vi "Main.vi"(10 "Monedas Subpanel":refnum<vi>, 11 "Module Admin":refnum<class "Delacor_lib_QMH_Module Admin.lvclass">) -> ()   [LabVIEW 2020, in "Monedas.lvlib"]
doc: "This template is based off of the Queued Message Handler design pattern and the Queued Message Handler project template that ships with LabVIEW.\n\nThe main difference is that the queue is private to this module and communication between modules is performed via Broadcast and Request events.\n\nRequest events are wrapped in public API methods and are handled in the Event Handling Loop (EHL) of this VI. Any module can register for Broadcast events sent by this module. The EHL generates messages based on user interface actions.\n\nThe Message Handling Loop (MHL) processes messages generated by the EHL, or by other messages. The messages are string values, so new messages can be added easily to the Message Cases case structure in the MHL. Each message cluster can also provide an optional value for Message Data, which is a variant that can be converted to whatever message-specific data is required.\n_____\nBased on Delacor QMH Project Template 5.0.0.82."
uses:
  Monedas.lvlib
  <vilib>/Delacor/Delacor QMH/Libraries/Module Admin_class/Delacor_lib_QMH_Module Admin.lvclass
  Module Data--cluster.ctl
  Type defMonedasread.ctl
  Stop Argument--cluster.ctl
  <vilib>/Delacor/Delacor QMH/Libraries/Message Queue_class/Delacor_lib_QMH_Message Queue.lvclass/Delacor_lib_QMH_Message Queue.ctl
  <vilib>/Delacor/Delacor QMH/Libraries/Module Admin_class/Delacor_lib_QMH_Module Admin.lvclass/Delacor_lib_QMH_Module Admin.ctl
  botones uno, dos, tres, cuatro Argument--cluster.ctl
  Set Coins Valuessssss Argument--cluster.ctl
  <vilib>/Utility/miscctls.llb/LVPointTypeDef.ctl
  <vilib>/Delacor/Delacor QMH/Libraries/Message Queue_class/Delacor_lib_QMH_Enqueue Message (Single).vi
  <vilib>/Delacor/Delacor QMH/Libraries/Module Admin_class/Delacor_lib_QMH_Get External Launch.vi
  <vilib>/Utility/error.llb/Error Cluster From Error Code.vi
  <vilib>/ErrorRing/Error Ring.xnode
  <vilib>/Delacor/Delacor QMH/Libraries/Message Queue_class/Delacor_lib_QMH_Message Queue.lvclass
  Mensajes/Mensajes.lvlib
  Config/Config.lvlib
  Producto/Producto.lvlib
panel:
  out "Valores monedas":dbl
  in  "Monedas cluster":T1
  out "error out":errorcluster
  out "Status":string
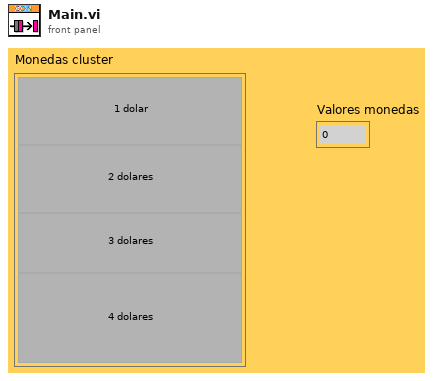
[diagram p1: front panel]
types:
  T1 = cluster{"1 cash":bool, "2 cash":bool, "3 cash":bool, "4 cash ":bool}
  T2 = typedef "Producto.lvlib/Broadcast Events--cluster.ctl" = cluster{"Module Did Init":refnum<user-event>, "Status Updated":refnum<user-event>, "Error Reported":refnum<user-event>, "Module Did Stop":refnum<user-event>, "Update Module Execution Status":refnum<user-event>}
  T3 = typedef "Mensajes.lvlib/Broadcast Events--cluster.ctl" = cluster{"Module Did Init":refnum<user-event>, "Status Updated":refnum<user-event>, "Error Reported":refnum<user-event>, "Module Did Stop":refnum<user-event>, "Update Module Execution Status":refnum<user-event>}
  T4 = typedef "Config.lvlib/Broadcast Events--cluster.ctl" = cluster{"Module Did Init":refnum<user-event>, "Status Updated":refnum<user-event>, "Error Reported":refnum<user-event>, "Module Did Stop":refnum<user-event>, "Update Module Execution Status":refnum<user-event>}
  T5 = typedef "Monedas.lvlib/Request Events--cluster.ctl" = cluster{"Stop Module":refnum<user-event>, "Show Panel":refnum<user-event>, "Hide Panel":refnum<user-event>, "Get Module Execution Status":refnum<user-event>, "Show Diagram":refnum<user-event>, "botones uno, dos, tres, cuatro":refnum<user-event>, "Set Coins Valuessssss":refnum<user-event>}
  T6 = typedef "Monedas.lvlib/Module Data--cluster.ctl" = cluster{"Status":string, "Coins":T7, "Monedas cluster":cluster{"1 cash":bool, "2 cash":bool, "3 cash":bool, "4 cash ":bool}, "Valores monedas":dbl, "refs":cluster{"Reference boton 1":refnum<vi>, "Reference boton 2":refnum<vi>, "Reference boton 3":refnum<vi>, "Reference boton 4":refnum<vi>}}
  T7 = typedef "Type defMonedasread.ctl" = cluster{"Boolean Text":string, "Value":dbl}[]
  T8 = enum32{"invalid lock state", "Not Locked", "Locked (No Password)", "Password-protected"}
  T9 = typedef "Monedas.lvlib/Stop Argument--cluster.ctl" = cluster{"Origin":string, "Exit via Stop Module Req?":bool, "Wait for Module to stop?":bool}
  T10 = typedef "Monedas.lvlib/botones uno, dos, tres, cuatro Argument--cluster.ctl" = cluster{"Monedas cluster":cluster{"1 cash":bool, "2 cash":bool, "3 cash":bool, "4 cash ":bool}}
  T11 = typedef "Monedas.lvlib/Set Coins Valuessssss Argument--cluster.ctl" = cluster{"COINS":cluster{"Boolean Text":string, "Numeric":dbl}[]}
  T12 = typedef "LVPointTypeDef.ctl" = cluster{"Horizontal":i16, "Vertical":i16}
  T13 = enum32{"Invalid", "Standard", "Closed", "Hidden", "Minimized", "Maximized"}
  T14 = cluster{"Reference boton 1":refnum<vi>, "Reference boton 2":refnum<vi>, "Reference boton 3":refnum<vi>, "Reference boton 4":refnum<vi>}
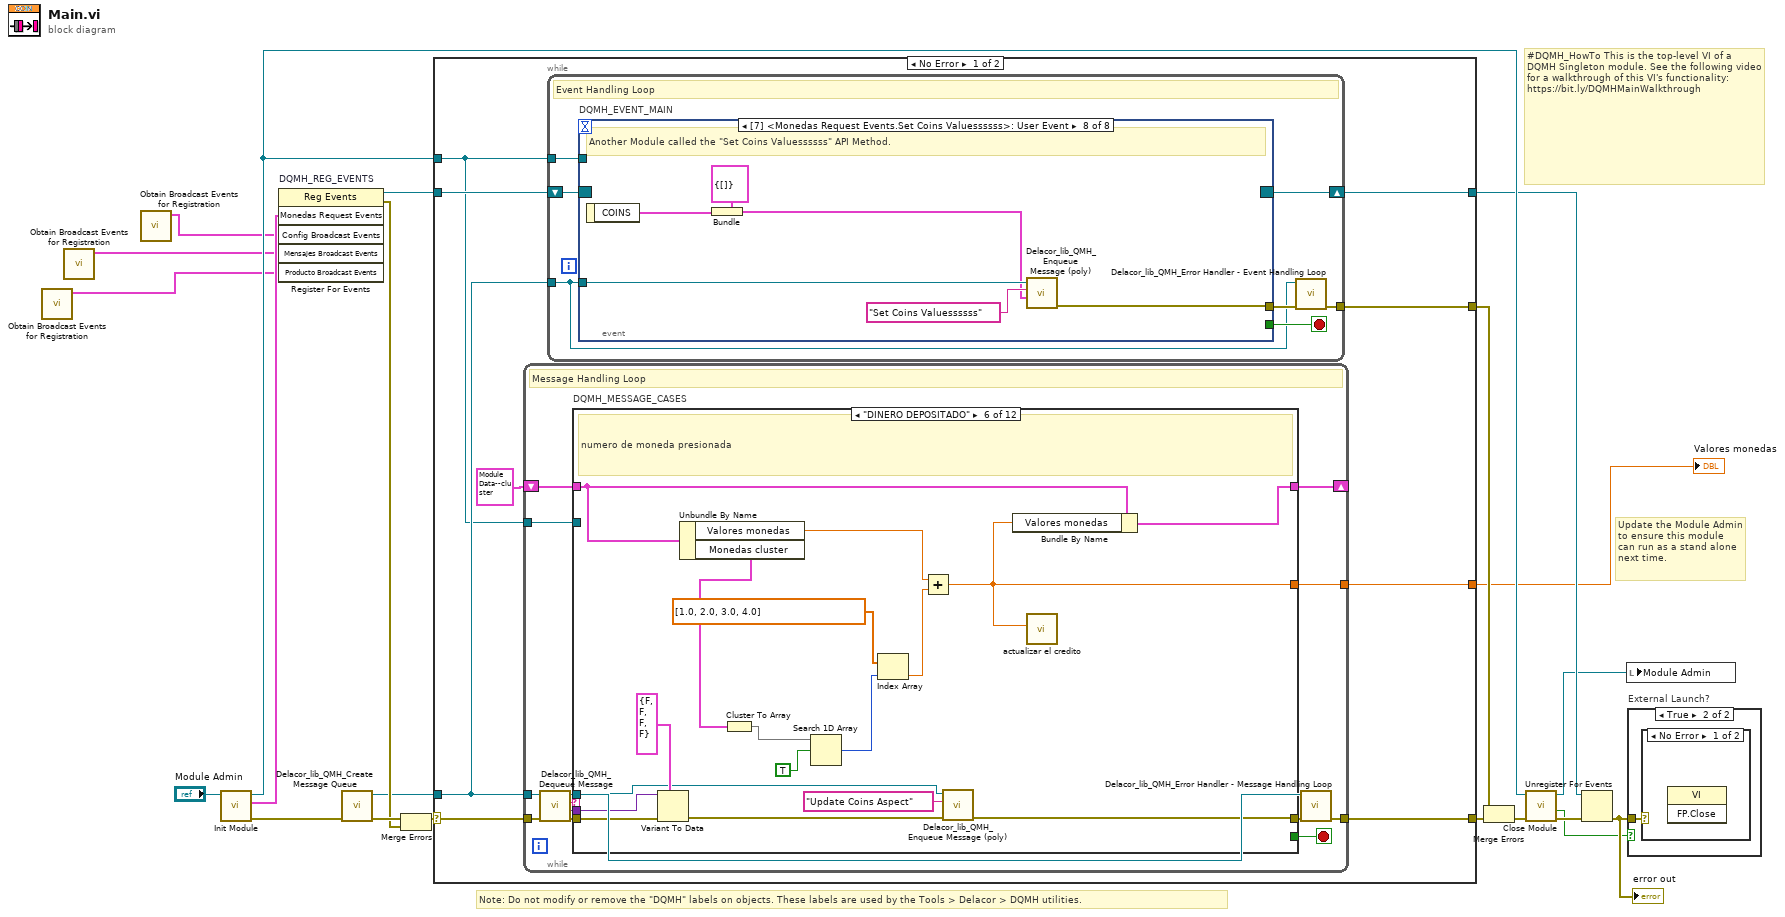
[diagram p0: block diagram]
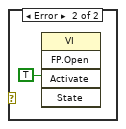
[diagram p3: hidden frame]
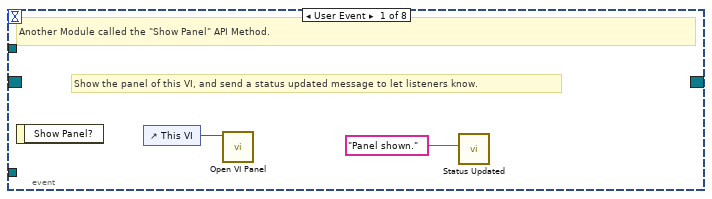
[diagram p4: hidden frame]
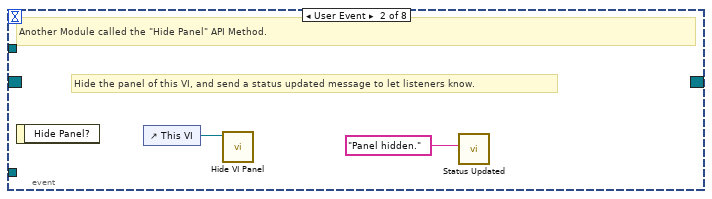
[diagram p5: hidden frame]
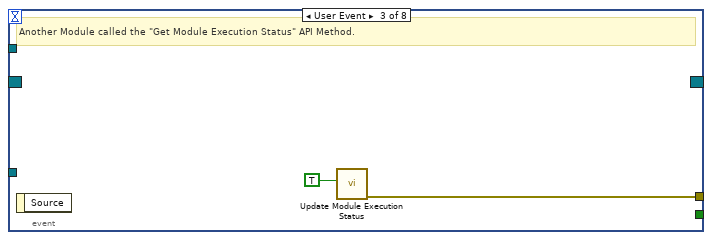
[diagram p6: hidden frame]
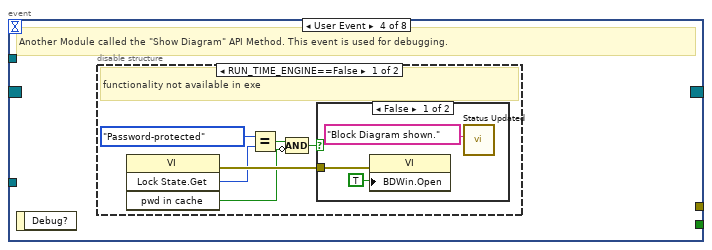
[diagram p7: hidden frame]
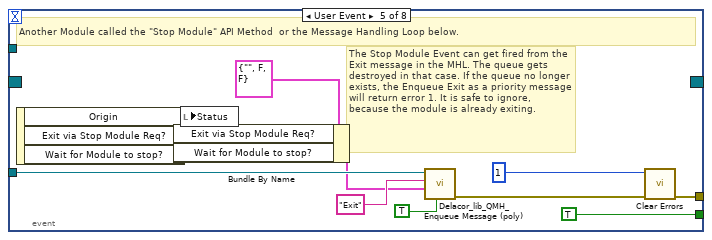
[diagram p10: hidden frame]
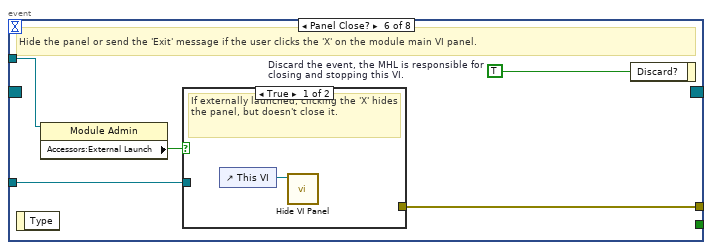
[diagram p11: hidden frame]
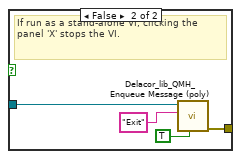
[diagram p12: hidden frame]
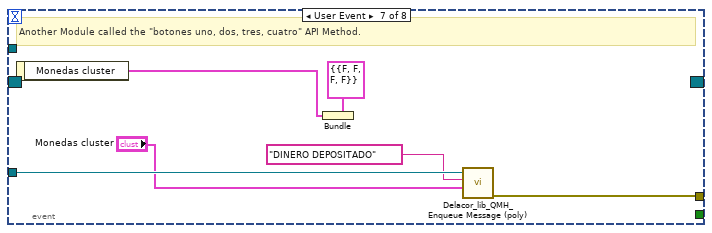
[diagram p13: hidden frame]
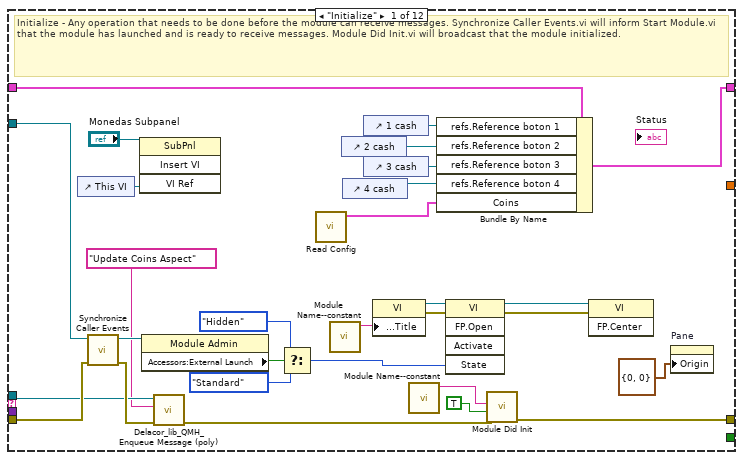
[diagram p14: hidden frame]
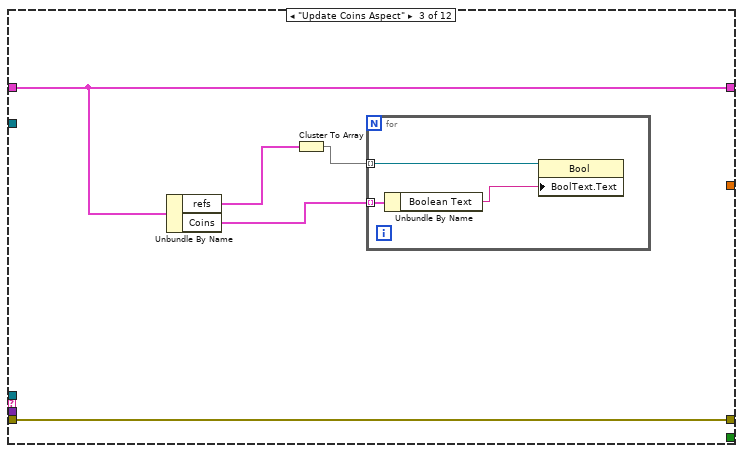
[diagram p16: hidden frame]
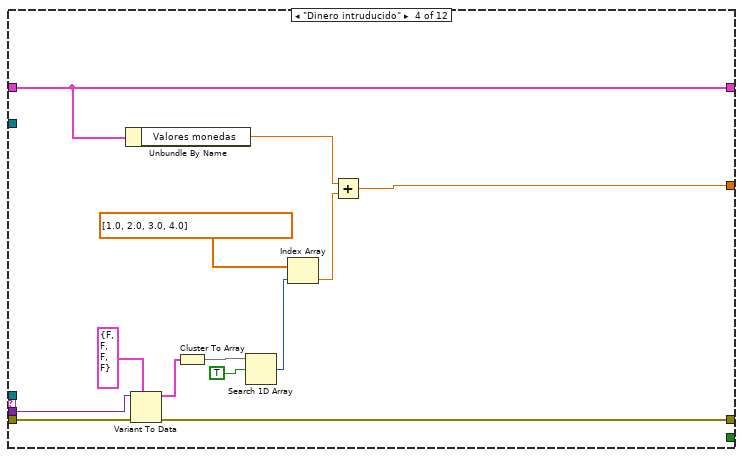
[diagram p17: hidden frame]
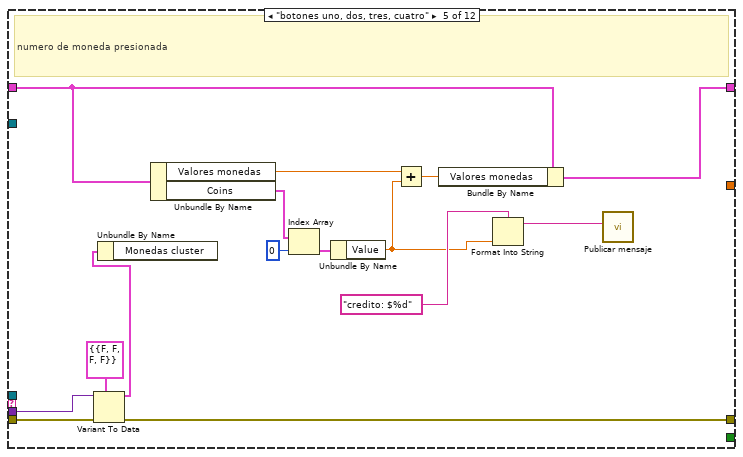
[diagram p18: hidden frame]
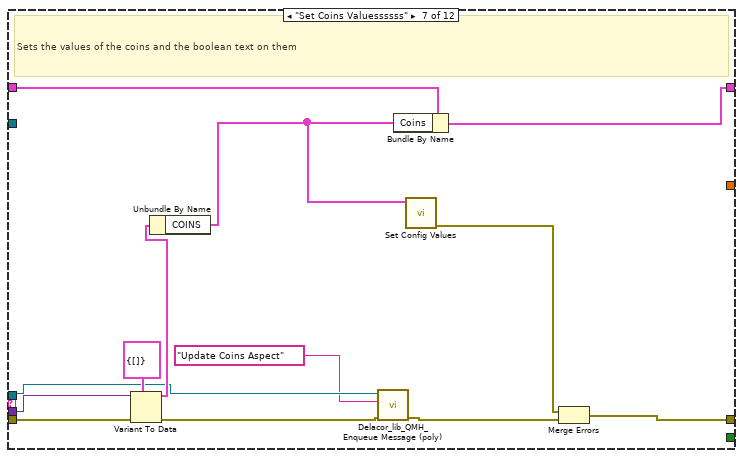
[diagram p19: hidden frame]
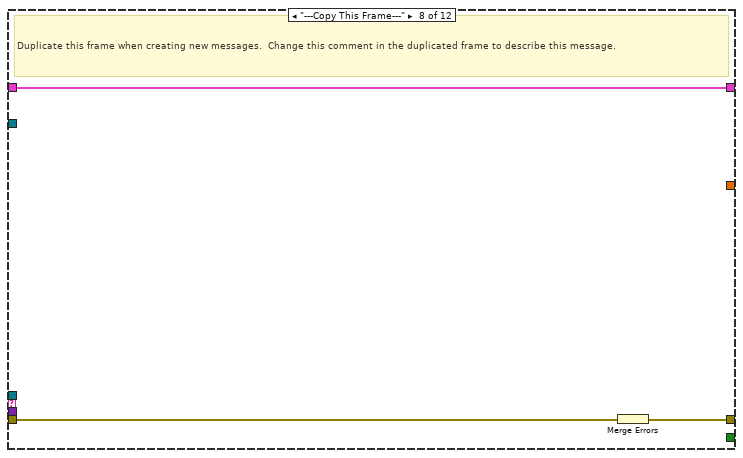
[diagram p20: hidden frame]
diagram:
  # "#DQMH_HowTo This is the top-level VI of a DQMH Singleton module. See the following video for a walkthrough of this VI's functionality: https://bit.ly/DQMHMainWalkthrough"
  # "Note: Do not modify or remove the \"DQMH\" labels on objects. These labels are used by the Tools > Delacor > DQMH utilities."
  # "Update the Module Admin to ensure this module can run as a stand alone next time."
  n1 = call "Obtain Broadcast Events for Registration.vi"() -> ("Producto Broadcast Events"=w1:T2)  [unwired: 9 in, 2 out]
  n2 = call "Obtain Broadcast Events for Registration.vi"() -> ("Mensajes Broadcast Events"=w2:T3)  [unwired: 9 in, 2 out]
  n3 = call "Obtain Broadcast Events for Registration.vi"() -> ("Config Broadcast Events"=w3:T4)  [unwired: 9 in, 2 out]
  n4 = call "Init Module.vi"("Singleton Module Admin in"="Module Admin") -> ("error out"=w20:errorcluster, "Monedas Request Events"=w9:T5, "Singleton Module Admin out"=w12:refnum<class "Delacor_lib_QMH_Module Admin.lvclass">)  [unwired: 8 in]
  n5 = register-events "DQMH_REG_EVENTS"(w9, w3, w2, w1) -> (reference out=w10:refnum<event-registration>, error out=w13:errorcluster)  [unwired: 2 in]
  n6 = call <vilib>:"Delacor_lib_QMH_Create Message Queue.vi"("error in (no error)"=w20) -> ("error out"=w15:errorcluster, "Message Queue"=w8:refnum<class "Delacor_lib_QMH_Message Queue.lvclass">)  [unwired: 9 in]
  n7 = Merge Errors(w15, w13) -> (w14:errorcluster)
  n8 = case shown="No Error" w14 {
    selector: w14 -> [w28 w250]
    tunnel: [w30 w249] -> w21
    tunnel: [w27 w255] -> w11
    tunnel: w10 -> [w25 w255]
    tunnel: w8 -> [w24 w248]
    tunnel: [w29 _] -> w18
    tunnel: w12 -> [w23 w251]
    tunnel: [w22 _] -> w4
    frame No Error {
      n9 = while {
        tunnel: w24 -> [w90]
        shift-right: [w94] -> _
        shift-left: T6 {"Status"="", "Coins"=[], "Monedas cluster"={"1 cash"=FALSE, "2 cash"=FALSE, "3 cash"=FALSE, "4 cash "=FALSE}, "Valores monedas"=0.0, "refs"={"Reference boton 1"=refnum, "Reference boton 2"=refnum, "Reference boton 3"=refnum, "Reference boton 4"=refnum}} ("Data Cluster") -> [w95]
        tunnel: w28 -> [w98]
        tunnel: [w96] -> w30
        tunnel: w23 -> [w88]
        tunnel: [w87] -> w22
        stop <- w93 stop-if-true
        # "Message Handling Loop"
        n10 = call-dynamic "Delacor_lib_QMH_Dequeue Message.vi"("error in (no error)"=w98, "Message Queue in"=w90) -> ("error out"=w97:errorcluster, "Message Data"=w91:variant, "Message"=w92:string, "Message Queue out"=w89:refnum<class "Delacor_lib_QMH_Message Queue.lvclass">)  [unwired: 6 in]
        n11 = case "DQMH_MESSAGE_CASES" shown="\"DINERO DEPOSITADO\"" w92 {
          selector: w92 -> [_ _ _ _ _ _ _ _ _ _ _ w235]
          tunnel: w89 -> [w101 _ _ _ _ w168 w187 _ _ w205 w227 _]
          tunnel: w97 -> [w126 w130 w135 w151 w166 w183 w196 w199 w201 w212 w233 w237]
          tunnel: [w104 w130 w135 w150 w155 w169 w185 w198 w201 w208 w230 w238] -> w99
          tunnel: w95 -> [w111 w129 w134 w142 w159 w174 w192 w197 w200 w207 w226 w236]
          tunnel: [w109 w129 w134 w142 w157 w173 w191 w197 w200 w207 w226 w236] -> w94
          tunnel: [_ _ _ _ _ _ _ _ _ _ w225 _] -> w93
          tunnel: w91 -> [_ _ _ w149 w165 w182 w195 _ _ w206 w224 _]
          tunnel: w88 -> [w118 _ _ _ _ _ _ _ _ w204 w219 _]
          tunnel: [_ _ _ w139 _ w172 _ _ _ _ _ _] -> w87
          frame "Initialize" {
            # "Initialize - Any operation that needs to be done before the module can receive messages. Synchronize Caller Events.vi will inform Start Module.vi that the module has launched and is ready to receive messages. Module Did Init.vi will broadcast that the module initialized."
            n12 = control-ref of="This VI"() -> (w112:refnum<vi>)
            n13 = call "Synchronize Caller Events.vi"("error in (no error)"=w126, "Singleton Module Admin in"=w118) -> ("error out"=w102:errorcluster, "Singleton Module Admin out"=w115:refnum<class "Delacor_lib_QMH_Module Admin.lvclass">)  [unwired: 8 in]
            n14 = invoke class="SubPnl" method="Insert VI"(reference="Monedas Subpanel", "VI Ref"=w112) -> ()  [unwired: 2 in, 4 out]
            n15 = property class="Module Admin"(reference=w115) -> ("Accessors:External Launch"=w122:bool)  [unwired: 1 in, 2 out]
            n16 = call-poly <vilib>:"Delacor_lib_QMH_Enqueue Message (poly).vi"("error in (no error)"=w102, "Message"="Update Coins Aspect", "Message Queue in"=w101) -> ("error out"=w103:errorcluster)  [unwired: 7 in, 1 out]
            n17 = Select(t=T13."Hidden" ("State"), s=w122, f=T13."Standard" ("State")) -> (s? t:f=w119:T13)
            n18 = call "Read Config.vi"() -> ("value"=w105:T7)  [unwired: 10 in, 1 out]
            n19 = call "Module Name--constant.vi"() -> ("Module Name"=w125:string)  [unwired: 11 in]
            n20 = control-ref of="2 cash"() -> (w108:refnum<vi>)
            n21 = control-ref of="4 cash"() -> (w106:refnum<vi>)
            n22 = control-ref of="1 cash"() -> (w110:refnum<vi>)
            n23 = control-ref of="3 cash"() -> (w107:refnum<vi>)
            n24 = property class="VI"("Front Panel.Title"=w125) -> (reference out=w124:refnum<vi>, error out=w128:errorcluster)  [unwired: 2 in]
            n25 = call "Module Name--constant.vi"() -> ("Module Name"=w116:string)  [unwired: 11 in]
            n26 = Bundle By Name(cluster=w111, "refs.Reference boton 1"=w110, "refs.Reference boton 2"=w108, "refs.Reference boton 3"=w107, "refs.Reference boton 4"=w106, "Coins"=w105) -> (w109:T6)
            n27 = invoke class="VI" method="FP.Open"(reference=w124, error in=w128, "State"=w119) -> (reference out=w123:refnum<vi>, error out=w127:errorcluster)  [unwired: 2 in, 3 out]
            n28 = call "Module Did Init.vi"("error in (no error)"=w103, "Initialized?"=TRUE, "Origin"=w116) -> ("error out"=w104:errorcluster)  [unwired: 8 in]
            n29 = invoke class="VI" method="FP.Center"(reference=w123, error in=w127) -> ()  [unwired: 1 in, 3 out]
            n30 = property on="Pane" class="Pane"("Origin"=T12 {"Horizontal"=0, "Vertical"=0}) -> ()  [unwired: 2 in, 2 out]
          }
          frame "--- Module Specific ---" {
            # "Separator -- The following cases handle messages specific to this Module."
          }
          frame "Update Coins Aspect" {
            n31 = Unbundle By Name(w134) -> ("refs"=w132:T14, "Coins"=w133:T7)
            n32 = Cluster To Array(cluster=w132) -> (array=w131:refnum<vi>[])
            n33 = for {
              tunnel: w133 -> [w138] mode=indexing
              tunnel: w131 -> [w137] mode=indexing
              n34 = Unbundle By Name(w138) -> ("Boolean Text"=w136:string)
              n35 = property class="Bool"(reference=w137, "BoolText.Text"=w136) -> ()  [unwired: 1 in, 2 out]
            }
          }
          frame "Dinero intruducido" {
            n36 = Unbundle By Name(w142) -> ("Valores monedas"=w140:dbl)
            n37 = Variant To Data(error in=w151, type=cluster{bool, bool, bool, bool} {FALSE, FALSE, FALSE, FALSE}, Variant=w149) -> (data=w145:cluster{bool, bool, bool, bool}, error out=w150:errorcluster)
            n38 = Cluster To Array(cluster=w145) -> (array=w144:bool[])
            n39 = Search 1D Array(1D array=w144, element=TRUE) -> (index of element=w146:i32)  [unwired: 1 in]
            n40 = Index Array "Index Array"(array=dbl[] [1.0, 2.0, 3.0, 4.0], index=w146) -> (element=w141:dbl)
            n41 = Add(x=w140, y=w141) -> (x+y=w139:dbl)
          }
          frame "botones uno, dos, tres, cuatro" {
            # "numero de moneda presionada"
            n42 = Variant To Data(error in=w166, type=T10 {"Monedas cluster"={"1 cash"=FALSE, "2 cash"=FALSE, "3 cash"=FALSE, "4 cash "=FALSE}} ("botones uno, dos, tres, cuatro Argument"), Variant=w165) -> (data=w163:T10, error out=w155:errorcluster)
            n43 = Unbundle By Name(w163) -> ()  [unwired: 1 out]
            n44 = Unbundle By Name(w159) -> ("Valores monedas"=w160:dbl, "Coins"=w162:T7)
            n45 = Index Array(array=w162, index=0) -> (element=w161:cluster{"Boolean Text":string, "Value":dbl})
            n46 = Unbundle By Name(w161) -> ("Value"=w154:dbl)
            n47 = Add(x=w160, y=w154) -> (x+y=w153:dbl)
            n48 = Bundle By Name(cluster=w159, "Valores monedas"=w153) -> (w157:T6)
            n49 = Format Into String(format string="credito: $%d", w154) -> (resulting string=w156:string)  [unwired: 2 in, 1 out]
            n50 = call "Publicar mensaje.vi"("Mensaje"=w156) -> ()  [unwired: 10 in, 1 out]
          }
          frame "DINERO DEPOSITADO" {
            # "numero de moneda presionada"
            n51 = Variant To Data(error in=w183, type=T1 {"1 cash"=FALSE, "2 cash"=FALSE, "3 cash"=FALSE, "4 cash "=FALSE} ("element"), Variant=w182) -> (error out=w170:errorcluster)  [unwired: 1 out]
            n52 = Unbundle By Name(w174) -> ("Valores monedas"=w181:dbl, "Monedas cluster"=w171:T1)
            n53 = Cluster To Array(cluster=w171) -> (array=w180:bool[])
            n54 = Search 1D Array(1D array=w180, element=TRUE) -> (index of element=w179:i32)  [unwired: 1 in]
            n55 = Index Array "Index Array"(array=dbl[] [1.0, 2.0, 3.0, 4.0], index=w179) -> (element=w177:dbl)
            n56 = Add(x=w181, y=w177) -> (x+y=w172:dbl)
            n57 = call-poly <vilib>:"Delacor_lib_QMH_Enqueue Message (poly).vi"("error in (no error)"=w170, "Message"="Update Coins Aspect", "Message Queue in"=w168) -> ("error out"=w169:errorcluster)  [unwired: 7 in, 1 out]
            n58 = Bundle By Name(cluster=w174, "Valores monedas"=w172) -> (w173:T6)
            n59 = call "actualizar el credito.vi"("Numeric"=w172) -> ()  [unwired: 10 in, 1 out]
          }
          frame "Set Coins Valuessssss" {
            # "Sets the values of the coins and the boolean text on them"
            n60 = Variant To Data(error in=w196, type=T11 {"COINS"=[]} ("Set Coins Valuessssss Argument"), Variant=w195) -> (data=w193:T11, error out=w189:errorcluster)
            n61 = Unbundle By Name(w193) -> ("COINS"=w190:cluster{"Boolean Text":string, "Numeric":dbl}[])
            n62 = call-poly <vilib>:"Delacor_lib_QMH_Enqueue Message (poly).vi"("error in (no error)"=w189, "Message"="Update Coins Aspect", "Message Queue in"=w187) -> ("error out"=w188:errorcluster)  [unwired: 7 in, 1 out]
            n63 = Bundle By Name(cluster=w192, "Coins"=w190) -> (w191:T6)
            n64 = call "Set Config Values.vi"("Coins"=w190) -> ("error out"=w184:errorcluster)  [unwired: 10 in]
            n65 = Merge Errors(w184, w188) -> (w185:errorcluster)
          }
          frame "---Copy This Frame---" {
            # "Duplicate this frame when creating new messages.  Change this comment in the duplicated frame to describe this message."
            n66 = Merge Errors(w199) -> (w198:errorcluster)
          }
          frame "--- Exit and Error Handling---" {
            # "Separator - The following cases handle errors and exit messages."
          }
          frame "Error" {
            # "#CodeRecommended - If you ever change the name of this \"Error\" message, you'll need to update the name in the Check Loop Error.vi as well."
            # "#CodeRecommended - If the module is running in standalone mode (External Launch = FALSE), this code will pop up an error dialog and call the 'Exit' message if an error occurs. Add more fine-grained error handling here."
            # "Error - Check the error message data and respond accordingly. This message is sent by the \"Error Handler\" VIs at the end of each loop in this application."
            n67 = property class="Module Admin"(reference=w204) -> ("Accessors:External Launch"=w203:bool)  [unwired: 1 in, 2 out]
            n68 = Variant To Data(error in=w212, type=errorcluster {"status"=FALSE, "code"=0, "source"=""} ("error constant"), Variant=w206) -> (data=w213:errorcluster, error out=w210:errorcluster)
            n69 = call "Module Name--constant.vi"() -> ("Module Name"=w202:string)  [unwired: 11 in]
            n70 = call "Error Reported.vi"("Additional Information"=w202, "Error"=w213) -> ()  [unwired: 9 in, 1 out]
            n71 = case shown="True" w203 {
              tunnel: [w218 _] -> w209
              tunnel: w205 -> [w216 _]
              tunnel: w213 -> [w217 _]
              frame False {
                # "If the module is running standalone, then pop up an error dialog and call the \"Exit\" message."
                n72 = call <vilib>:"Simple Error Handler.vi"("error in (no error)"=w217) -> ()  [unwired: 4 in, 5 out]
                n73 = call-poly <vilib>:"Delacor_lib_QMH_Enqueue Message (poly).vi"("Priority Message? (F)"=TRUE, "Message"="Exit", "Message Queue in"=w216) -> ("error out"=w218:errorcluster)  [unwired: 7 in, 1 out]
              }
              frame True {
                # "If the module was launched externally, calling the Error Reported broadcast VI is the only action performed by the \"Error\" message. The module's caller can then process the error appropriately."
              }
            }
            n74 = Merge Errors(w210, w209) -> (w208:errorcluster)
            n75 = local write "error out"(w208) -> ()
          }
          frame "Exit" {
            w223 = 91  # 91: not all Exit messages will have an argument
            w225 = TRUE  # Stop the VI
            # "Release the message queue reference"
            # "#CodeNeeded - Add any required cleanup code here"
            # "Exit - Exit the application."
            n76 = Variant To Data(error in=w233, type=T9 {"Origin"="", "Exit via Stop Module Req?"=FALSE, "Wait for Module to stop?"=FALSE} ("Stop Argument"), Variant=w224) -> (data=w221:T9, error out=w229:errorcluster)
            n77 = call <vilib>:"Clear Errors.vi"("error in (no error)"=w229, "specific error code to clear (0: all)"=w223) -> ("error out"=w232:errorcluster)  [unwired: 4 in, 1 out]
            n78 = control-ref of="This VI"() -> (w220:refnum<vi>)
            n79 = call-dynamic "Delacor_lib_QMH_Release Message Queue.vi"("error in (no error)"=w232, "Message Queue"=w227) -> ("error out"=w231:errorcluster)  [unwired: 9 in]
            n80 = call "Handle Exit.vi"("Stop Argument"=w221, "Admin in"=w219, "VI reference"=w220) -> ("error out"=w228:errorcluster)  [unwired: 7 in, 1 out]
            n81 = Merge Errors(w231, w228) -> (w230:errorcluster)
          }
          frame Default {
            # "'Default' case only runs if there is a message that isn't defined in any of the other cases.  Output a programming error."
            n82 = call "Module Name--constant.vi"() -> ("Module Name"=w234:string)  [unwired: 11 in]
            n83 = xnode "Error Ring"("parameter 0"=w235, "parameter 1"=w234) -> ("error out"=w239:errorcluster)
            n84 = Merge Errors(w237, w239) -> (w238:errorcluster)
          }
        }
        n85 = call-dynamic "Delacor_lib_QMH_Error Handler - Message Handling Loop.vi"("error in (no error)"=w99, "Message Queue in"=w89) -> ("dup error in"=w96:errorcluster)  [unwired: 8 in, 1 out]
      }
      n86 = while {
        tunnel: w24 -> [w31]
        shift-right: [w34] -> w27
        shift-left: w25 -> [w35]
        tunnel: [w36] -> w29
        tunnel: w23 -> [w32]
        stop <- w33 stop-if-true
        # "Event Handling Loop"
        n87 = event "DQMH_EVENT_MAIN" shown="[7] <Monedas Request Events.Set Coins Valuessssss>: User Event" {
          selector: w35 -> [_ _ _ _ _ _ _ _]
          dyn-events: [_ _ _ _ _ _ _ _] -> w34
          timeout: _ -> [_ _ _ _ _ _ _ _]
          tunnel: [_ _ _ _ TRUE ("Discard?") _ _ _] -> w33
          tunnel: w31 -> [_ _ _ _ w60 w67 w80 w86]
          tunnel: [_ _ w43 _ w63 w69 w77 w81] -> w37
          tunnel: w32 -> [_ _ _ _ _ w66 _ _]
          event User Event {
            # "Show the panel of this VI, and send a status updated message to let listeners know."
            # "Another Module called the \"Show Panel\" API Method."
            n88 = event-data() -> ()  [unwired: 1 in, 1 out]
            n89 = control-ref of="This VI"() -> (w39:refnum<vi>)
            n90 = call "Open VI Panel.vi"("VI"=w39) -> ()  [unwired: 10 in, 1 out]
            n91 = call "Status Updated.vi"("Status"="Panel shown." ("format string")) -> ()  [unwired: 10 in, 1 out]
          }
          event User Event {
            # "Hide the panel of this VI, and send a status updated message to let listeners know."
            # "Another Module called the \"Hide Panel\" API Method."
            n92 = event-data() -> ()  [unwired: 1 in, 1 out]
            n93 = control-ref of="This VI"() -> (w41:refnum<vi>)
            n94 = call "Hide VI Panel.vi"("VI"=w41) -> ()  [unwired: 10 in, 1 out]
            n95 = call "Status Updated.vi"("Status"="Panel hidden." ("format string")) -> ()  [unwired: 10 in, 1 out]
          }
          event User Event {
            # "Another Module called the \"Get Module Execution Status\" API Method."
            n96 = event-data() -> ()  [unwired: 1 in, 1 out]
            n97 = call "Update Module Execution Status.vi"("Running?"=TRUE) -> ("error out"=w43:errorcluster)  [unwired: 10 in]
          }
          event User Event {
            # "Another Module called the \"Show Diagram\" API Method. This event is used for debugging."
            n98 = event-data() -> ()  [unwired: 1 in, 1 out]
            n99 = disable-structure shown="RUN_TIME_ENGINE==False" {
              frame condition #0 (active) {
                # "functionality not available in exe"
                n100 = invoke class="VI" method="Lock State.Get"() -> (error out=w49:errorcluster, "Get Lock State"=w48:T8, "pwd in cache"=w45:bool)  [unwired: 4 in, 1 out]
                n101 = Equal?(x=T8."Password-protected", y=w48) -> (x = y?=w46:bool)
                n102 = Compound Arithmetic op=AND(w46, invert w45) -> (w44:bool)
                n103 = case shown="False" w44 {
                  tunnel: w49 -> [w52 _]
                  frame False {
                    n104 = property class="VI"(error in=w52, "BDWin.Open"=TRUE ("Block Diagram Window:Open")) -> ()  [unwired: 1 in, 2 out]
                    n105 = call "Status Updated.vi"("Status"="Block Diagram shown." ("format string")) -> ()  [unwired: 10 in, 1 out]
                  }
                  frame True {
                    # "Password-protected VI, and the password is not in the cache. Do not show the diagram."
                  }
                }
              }
              frame condition #1 {
              }
            }
          }
          event User Event {
            # "The Stop Module Event can get fired from the Exit message in the MHL. The queue gets destroyed in that case. If the queue no longer exists, the Enqueue Exit as a priority message will return error 1. It is safe to ignore, because the module is already exiting."
            # "Another Module called the \"Stop Module\" API Method  or the Message Handling Loop below."
            n106 = event-data() -> ("Origin"=w59:string, "Exit via Stop Module Req?"=w55:bool, "Wait for Module to stop?"=w54:bool)  [unwired: 1 in]
            n107 = Bundle By Name(cluster=T9 {"Origin"="", "Exit via Stop Module Req?"=FALSE, "Wait for Module to stop?"=FALSE} ("Stop Argument"), "Exit via Stop Module Req?"=w55, "Wait for Module to stop?"=w54) -> (w53:T9)
            n108 = local write "Status"(w59) -> ()
            n109 = call-poly <vilib>:"Delacor_lib_QMH_Enqueue Message (poly).vi"("Priority Message? (F)"=TRUE, "Message Data"=w53, "Message"="Exit", "Message Queue in"=w60) -> ("error out"=w64:errorcluster)  [unwired: 6 in, 1 out]
            n110 = call <vilib>:"Clear Errors.vi"("error in (no error)"=w64, "specific error code to clear (0: all)"=1) -> ("error out"=w63:errorcluster)  [unwired: 4 in, 1 out]
          }
          event Panel Close? {
            w68 = TRUE  # Discard the event, the MHL is responsible for closing and stopping this VI.
            # "Hide the panel or send the 'Exit' message if the user clicks the 'X' on the module main VI panel."
            n111 = event-data() -> ()  [unwired: 1 in, 1 out]
            n112 = property class="Module Admin"(reference=w66) -> ("Accessors:External Launch"=w65:bool)  [unwired: 1 in, 2 out]
            n113 = case shown="True" w65 {
              tunnel: w67 -> [_ w73]
              tunnel: [_ w74] -> w69
              frame True {
                # "If externally launched, clicking the 'X' hides the panel, but doesn't close it."
                n114 = control-ref of="This VI"() -> (w70:refnum<vi>)
                n115 = call "Hide VI Panel.vi"("VI"=w70) -> ()  [unwired: 10 in, 1 out]
              }
              frame False {
                # "If run as a stand-alone VI, clicking the panel 'X' stops the VI."
                n116 = call-poly <vilib>:"Delacor_lib_QMH_Enqueue Message (poly).vi"("Priority Message? (F)"=TRUE, "Message"="Exit", "Message Queue in"=w73) -> ("error out"=w74:errorcluster)  [unwired: 7 in, 1 out]
              }
            }
            n117 = event-data("Discard?"=w68) -> ()  [unwired: 1 in, 1 out]
          }
          event User Event {
            # "Another Module called the \"botones uno, dos, tres, cuatro\" API Method."
            n118 = event-data() -> ("Monedas cluster"=w76:T1)  [unwired: 1 in]
            n119 = Bundle(cluster=T10 {"Monedas cluster"={"1 cash"=FALSE, "2 cash"=FALSE, "3 cash"=FALSE, "4 cash "=FALSE}} ("botones uno, dos, tres, cuatro Argument"), "Monedas cluster"=w76) -> ()  [unwired: 1 out]
            n120 = call-poly <vilib>:"Delacor_lib_QMH_Enqueue Message (poly).vi"("Message Data"="Monedas cluster", "Message"="DINERO DEPOSITADO", "Message Queue in"=w80) -> ("error out"=w77:errorcluster)  [unwired: 7 in, 1 out]
          }
          event User Event {
            # "Another Module called the \"Set Coins Valuessssss\" API Method."
            n121 = event-data() -> ("COINS"=w82:cluster{"Boolean Text":string, "Numeric":dbl}[])  [unwired: 1 in]
            n122 = Bundle(cluster=T11 {"COINS"=[]} ("Set Coins Valuessssss Argument"), "COINS"=w82) -> (w83:T11)
            n123 = call-poly <vilib>:"Delacor_lib_QMH_Enqueue Message (poly).vi"("Message Data"=w83, "Message"="Set Coins Valuessssss", "Message Queue in"=w86) -> ("error out"=w81:errorcluster)  [unwired: 7 in, 1 out]
          }
        }
        n124 = call-dynamic "Delacor_lib_QMH_Error Handler - Event Handling Loop.vi"("error in (no error)"=w37, "Message Queue in"=w31) -> ("dup error in"=w36:errorcluster)  [unwired: 8 in, 1 out]
      }
    }
    frame Error {
      # "Synchronize Caller Events.vi will inform Start Module.vi that the module has launched and will let the code calling Start Module.vi register for broadcasts and would permit the caller receive the broadcast that an error occurred at launch time."
      n125 = call-dynamic "Delacor_lib_QMH_Release Message Queue.vi"("error in (no error)"=w250, "Message Queue"=w248) -> ("error out"=w249:errorcluster)  [unwired: 9 in]
      n126 = call "Synchronize Caller Events.vi"("Singleton Module Admin in"=w251) -> ("error out"=w256:errorcluster)  [unwired: 9 in, 1 out]
      n127 = call "Module Name--constant.vi"() -> ("Module Name"=w254:string)  [unwired: 11 in]
      n128 = Format Into String(format string="An error occurred during initialization. %s is no longer running.", w254) -> (resulting string=w252:string)  [unwired: 2 in, 1 out]
      n129 = Merge Errors(w249, w256) -> (w257:errorcluster)
      n130 = call "Error Reported.vi"("Additional Information"=w252, "Error"=w257) -> ()  [unwired: 9 in, 1 out]
    }
  }
  "Valores monedas" <- w4
  n131 = Merge Errors(w18, w21) -> (w17:errorcluster)
  n132 = call "Close Module.vi"("error in (no error)"=w17, "Module Admin in"=w12) -> ("error out"=w19:errorcluster, "External Launch"=w5:bool, "Module Admin out"=w6:refnum<class "Delacor_lib_QMH_Module Admin.lvclass">)  [unwired: 7 in]
  n133 = Unregister For Events(event registration refnum=w11, error in=w19) -> (error out=w16:errorcluster)
  "error out" <- w16
  n134 = local write "Module Admin"(w6) -> ()
  n135 = case "External Launch?" shown="True" w5 {
    tunnel: w16 -> [_ w258]
    frame False {
    }
    frame True {
      n136 = case shown="No Error" w258 {
        frame No Error {
          n137 = invoke class="VI" method="FP.Close"() -> ()  [unwired: 3 in, 3 out]
        }
        frame Error {
          n138 = invoke class="VI" method="FP.Open"("Activate"=TRUE ("Activate?")) -> ()  [unwired: 4 in, 5 out]
        }
      }
    }
  }
